vi "SetCurrent(Basic).vi"(7 "Memory":i8=1 min=1 max=50, 8 "Error In":errorcluster, 10 "Current":dbl min=0.0 max=10.0 format="%.2g", 11 "VISA resource name":refnum<visa-resource-name>) -> (0 "Error Out":errorcluster, 3 "VISA resource name out":refnum<visa-resource-name>)   [LabVIEW 2013]
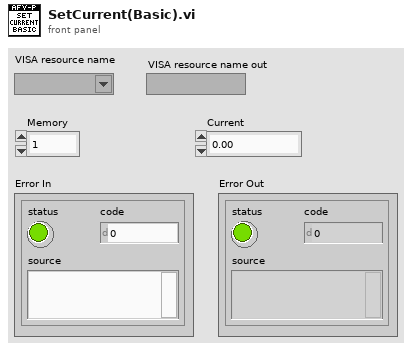
[diagram p1: front panel]
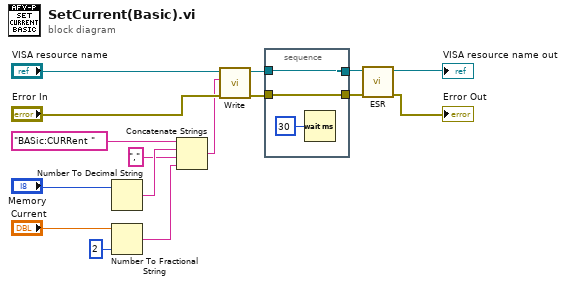
[diagram p0: block diagram]
diagram:
  n1 = Number To Decimal String(number="Memory") -> (decimal integer string=w9:string)  [unwired: 1 in]
  n2 = Number To Fractional String(number="Current", precision (6)=i16 2) -> (F-format string=w8:string)  [unwired: 2 in]
  n3 = Concatenate Strings("BASic:CURRent " ("Write Buffer"), w9, "," ("string"), w8) -> (w11:string)
  n4 = call "Write.vi"("Error In"="Error In", "Write Buffer"=w11, "VISA resource name"="VISA resource name") -> ("Error Out"=w3:errorcluster, "VISA resource name out"=w4:refnum<visa-resource-name>)  [unwired: 7 in]
  n5 = stacked-sequence {
    tunnel: [w18] -> w6
    tunnel: w4 -> [w18]
    tunnel: [w17] -> w5
    tunnel: w3 -> [w17]
    frame #0 {
      n6 = Wait (ms)(milliseconds to wait=u32 30) -> ()  [unwired: 1 out]
    }
  }
  n7 = call "ESR.vi"("Error In"=w5, "VISA resource name"=w6) -> ("Error Out"=→"Error Out":errorcluster, "VISA resource name out"=→"VISA resource name out":refnum<visa-resource-name>)  [unwired: 8 in]
